vi "All stations name config.vi"(7 "stations count":i32, 10 "station idx":i32, 11 "configuration file path":path) -> (0 "error out":errorcluster caption="错误输出", 2 "station idx":i32, 3 "configuration file path":path, 5 "station msic":T1)   [LabVIEW 2018]
uses:
  Crl defs/one state msic config.ctl
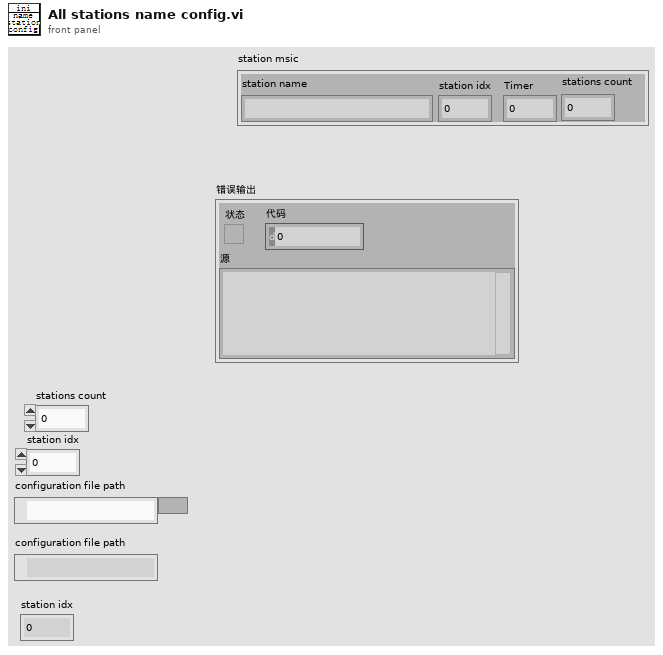
[diagram p1: front panel]
types:
  T1 = typedef "one state msic config.ctl" = cluster{"station name":string, "Timer":u32, "station idx":i32, "stations count":i32}
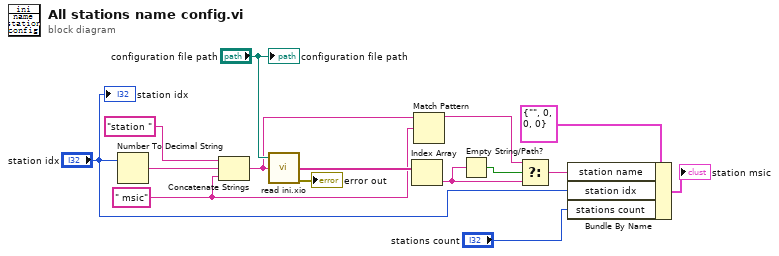
[diagram p0: block diagram]
diagram:
  w3 = " msic" ("string")
  n1 = Number To Decimal String(number="station idx") -> (decimal integer string=w13:string)  [unwired: 1 in]
  n2 = Concatenate Strings("station ", w13, w3) -> (w7:string)
  n3 = call "read ini.xio.vi"("configuration file path"="configuration file path", "Sections"=w7) -> ("Values"=w11:string[], "error out"=→"error out":errorcluster)  [unwired: 1 in, 3 out]
  n4 = Index Array(array=w11) -> (element=w5:string)  [unwired: 1 in]
  n5 = Match Pattern(string=w7, regular expression=w3) -> (before substring=w6:string)  [unwired: 1 in, 3 out]
  n6 = Empty String/Path?(string/path=w5) -> (empty?=w8:bool)
  n7 = Select(t=w6, s=w8, f=w5) -> (s? t:f=w4:string)
  n8 = Bundle By Name(cluster=T1 {"station name"="", "Timer"=0, "station idx"=0, "stations count"=0} ("station msic"), "station name"=w4, "station idx"="station idx", "stations count"="stations count") -> (→"station msic":T1)
  "configuration file path" <- "configuration file path"
  "station idx" <- "station idx"
